vi "DOCK_MAIN_get_reload_data.vi"(8 "error_in":errorcluster, 11 "variable":variant) -> (0 "error_out":errorcluster, 3 "reload_data":T1)   [LabVIEW 2019]
uses:
  ini/typedef/DOCK_reload_data.ctl
  _misc/AULocalize/SubVIs/Get Localized Phrase Compact Interface 0D.vi
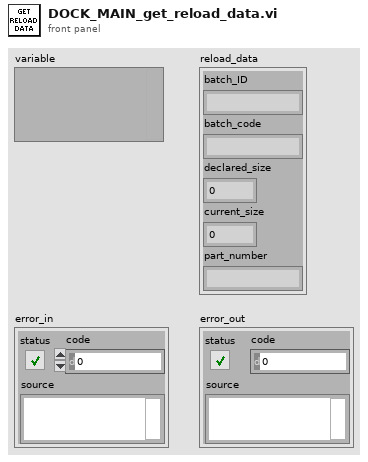
[diagram p1: front panel]
types:
  T1 = typedef "DOCK_reload_data.ctl" = cluster{"batch_ID":string, "batch_code":string, "declared_size":u16, "current_size":u16, "part_number":string}
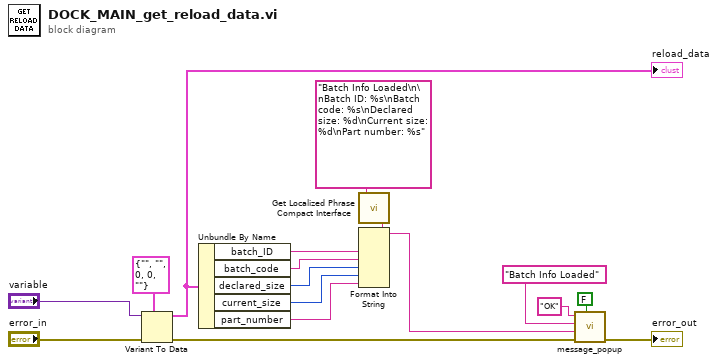
[diagram p0: block diagram]
diagram:
  n1 = Variant To Data(error in="error_in", type=T1 {"batch_ID"="", "batch_code"="", "declared_size"=0, "current_size"=0, "part_number"=""} ("reload_data"), Variant="variable") -> (data=w6:T1, error out=w3:errorcluster)
  "reload_data" <- w6
  n2 = Unbundle By Name(w6) -> ("batch_ID"=w7:string, "batch_code"=w8:string, "declared_size"=w9:u16, "current_size"=w10:u16, "part_number"=w11:string)
  n3 = call-poly "Get Localized Phrase Compact Interface.vi"("Key"="Batch Info Loaded\n\nBatch ID: %s\nBatch code: %s\nDeclared size: %d\nCurrent size: %d\nPart number: %s") -> ("Translated Phrase"=w1:string)
  n4 = Format Into String(format string=w1, w7, w8, w9, w10, w11) -> (resulting string=w16:string)  [unwired: 2 in, 1 out]
  n5 = call "message_popup.vi"("Warning(T)/Info(F)"=FALSE, "error_in"=w3, "Message"=w16, "Title"="Batch Info Loaded", "Button Label"="OK") -> ("error_out"=→"error_out":errorcluster)  [unwired: 6 in]
